vi "subVI QCam Load File Parameters.vi"() -> (0 "Ratio RedGreen":dbl, 1 "Ratio BlueGreen":dbl, 2 "exposure":dbl, 3 "exposure Red":dbl, 4 "exposure Blue":dbl)   [LabVIEW 2012]
panel:
  out "exposure64Blue":string
  out "exposure64Red":string
  out "exposure64":string
  out "File String":string
  # "Output"
  # "Input"
  # "Internal Variables"
  # "None"
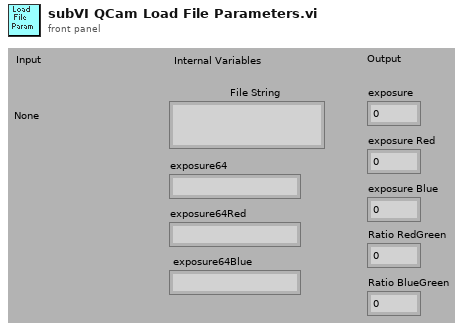
[diagram p1: front panel]
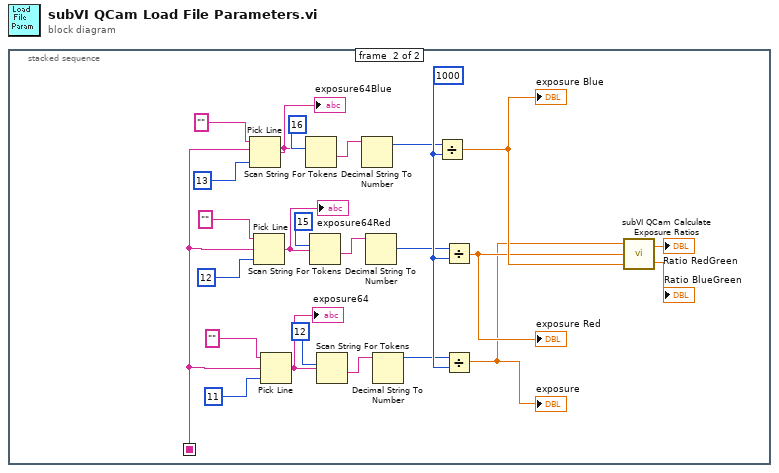
[diagram p0: block diagram]
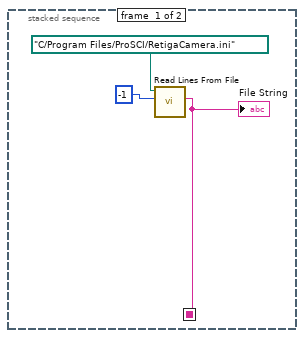
[diagram p2: hidden frame]
diagram:
  n1 = stacked-sequence {
    seq-local: [w1 _] -> [_ w9]
    frame #0 {
      n2 = call <vilib>:"Read Lines From File.vi"("file path (dialog if empty)"=path "C:/Program Files/ProSCI/RetigaCamera.ini", "number of lines (all:-1)"=-1) -> ("line string"=w1:string)  [unwired: 7 out]
      "File String" <- w1
    }
    frame #1 {
      w13 = 1000
      n3 = Pick Line(string ("")="", multi-line string=w9, line index=13) -> (output string=w14:string)
      "exposure64Blue" <- w14
      n4 = Pick Line(string ("")="", multi-line string=w9, line index=12) -> (output string=w15:string)
      "exposure64Red" <- w15
      n5 = Pick Line(string ("")="", multi-line string=w9, line index=11) -> (output string=w16:string)
      "exposure64" <- w16
      n6 = Scan String For Tokens(8:16 ("offset"), 9:w14) -> (1:w17:string)  [unwired: 7 out]
      n7 = Scan String For Tokens(8:15 ("offset"), 9:w15) -> (1:w21:string)  [unwired: 7 out]
      n8 = Scan String For Tokens(8:12 ("offset"), 9:w16) -> (1:w25:string)  [unwired: 7 out]
      n9 = Decimal String To Number(string=w17) -> (number=w12:i32)  [unwired: 3 out]
      n10 = Decimal String To Number(string=w21) -> (number=w11:i32)  [unwired: 3 out]
      n11 = Decimal String To Number(string=w25) -> (number=w10:i32)  [unwired: 3 out]
      n12 = Divide(x=w12, y=w13) -> (x/y=w6:dbl)
      "exposure Blue" <- w6
      n13 = Divide(x=w11, y=w13) -> (x/y=w5:dbl)
      "exposure Red" <- w5
      n14 = Divide(x=w10, y=w13) -> (x/y=w4:dbl)
      "exposure" <- w4
      n15 = call "subVI QCam Calculate Exposure Ratios.vi"("exposure Blue"=w6, "exposure Red"=w5, "exposure"=w4) -> ("Ratio BlueGreen"=→"Ratio BlueGreen":dbl, "Ratio RedGreen"=→"Ratio RedGreen":dbl)
    }
  }
